vi "ColourROIPicker.vi"() -> ()   [LabVIEW 2021]
uses:
  <vilib>/userDefined/High Color/IMAQdx.ctl
  <vilib>/vision/driver/IMAQdx.llb/IMAQdx Camera Control Mode.ctl
  <vilib>/vision/driver/IMAQdx.llb/IMAQdx Acquisition Mode.ctl
  <vilib>/vision/driver/IMAQdx.llb/IMAQdx Buffer Number Mode.ctl
  <vilib>/vision/driver/NI_Vision_Acquisition_Software.lvlib
  <resource>/objmgr/imaqdx.rc
  <vilib>/vision/NI_Vision_Development_Module.lvlib
panel:
  out "Is Colour from Sample Detected":bool
  out "Colour at Pixel Box":u32(colorbox)
  out "Colour at Pixel Value":u32
  out "Model":string
  out "Attr":T1(array[cluster]) caption="Camera Attributes"
  out "Image":T2(plugin-control)
  in  "Stop":bool
  out "error out":errorcluster
  # "RPV Test Rig 2024"
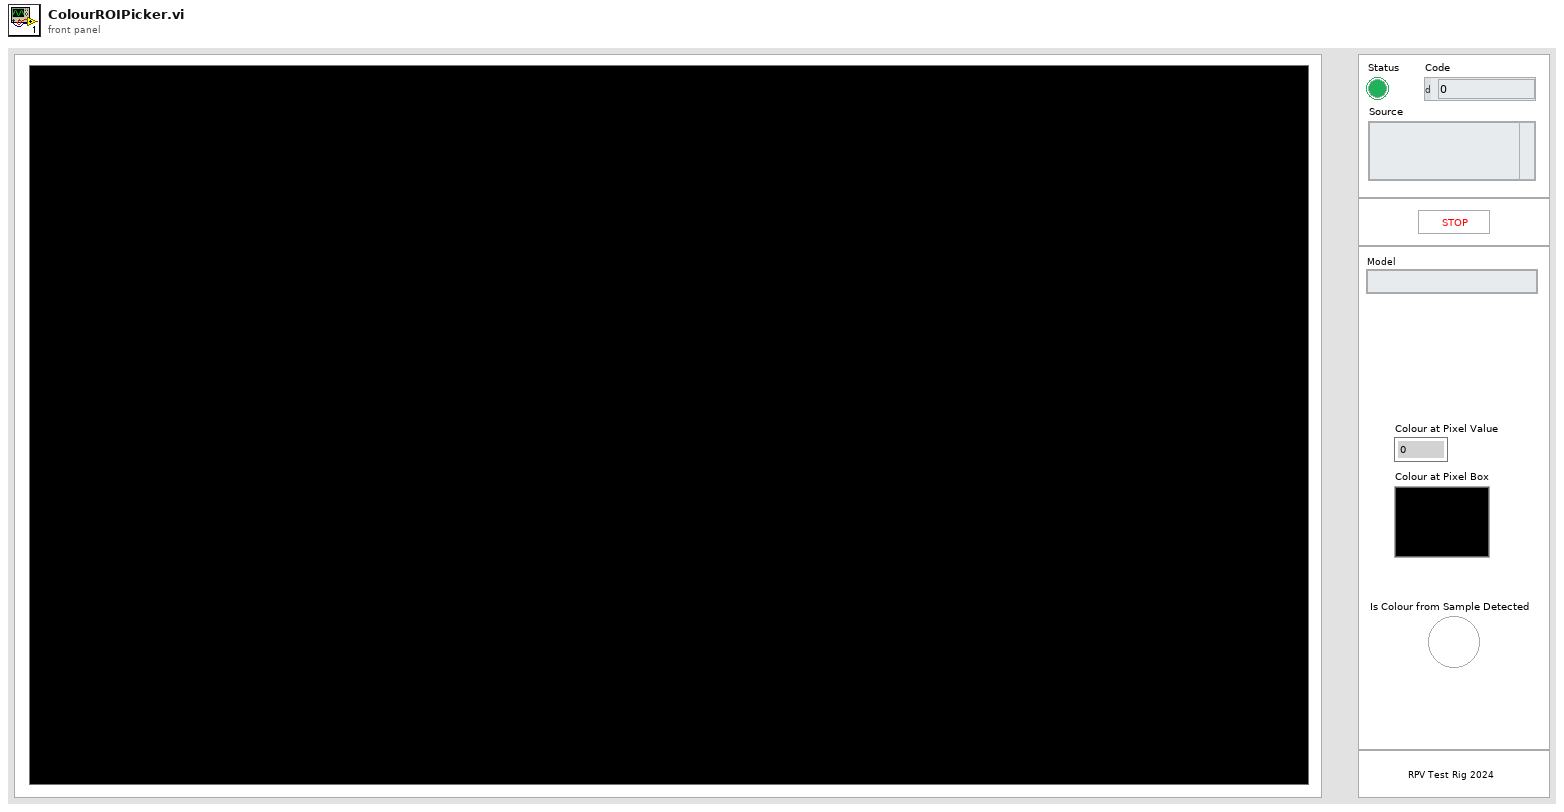
[diagram p1: front panel]
types:
  T1 = cluster{"Data Type":enum32{"U32", "I64", "DBL", "String", "Enum", "Bool", "Command"}, "Readable":bool, "Writable":bool, "Attribute Name":string}[]
  T2 = typedef "IMAQ Image.ctl" = refnum<image>
  T3 = typedef "IMAQ Rectangle" = cluster{"Left":i32, "Top":i32, "Right":i32, "Bottom":i32, "Rotation":dbl}
  T4 = typedef "NI_Vision_Acquisition_Software.lvlib/IMAQdx Buffer Number Mode.ctl" = enum32{"Next", "Last", "Buffer Number", "Every", "Last New"}
  T5 = typedef "NI_Vision_Acquisition_Software.lvlib/IMAQdx Acquisition Mode.ctl" = enum32{"One Shot", "Continuous"}
  T6 = typedef "NI_Vision_Acquisition_Software.lvlib/IMAQdx Camera Control Mode.ctl" = enum32{"Controller", "Listener"}
  T7 = typedef "IMAQdx.ctl" = refnum<k21>
  T8 = typedef "ROI Descriptor" = cluster{"Global Rectangle":i32[], "Contours":cluster{"ID":enum32{"External", "Internal"}, "Type":u32, "Coordinates":i32[]}[]}
  T9 = typedef "NI_Vision_Acquisition_Software.lvlib/IMAQdx Attribute Type.ctl" = enum32{"U32", "I64", "DBL", "String", "Enum", "Bool", "Command"}
  T10 = cluster{"Attribute Type":T9, "Readable":bool, "Writable":bool, "Attribute Name":string}[]
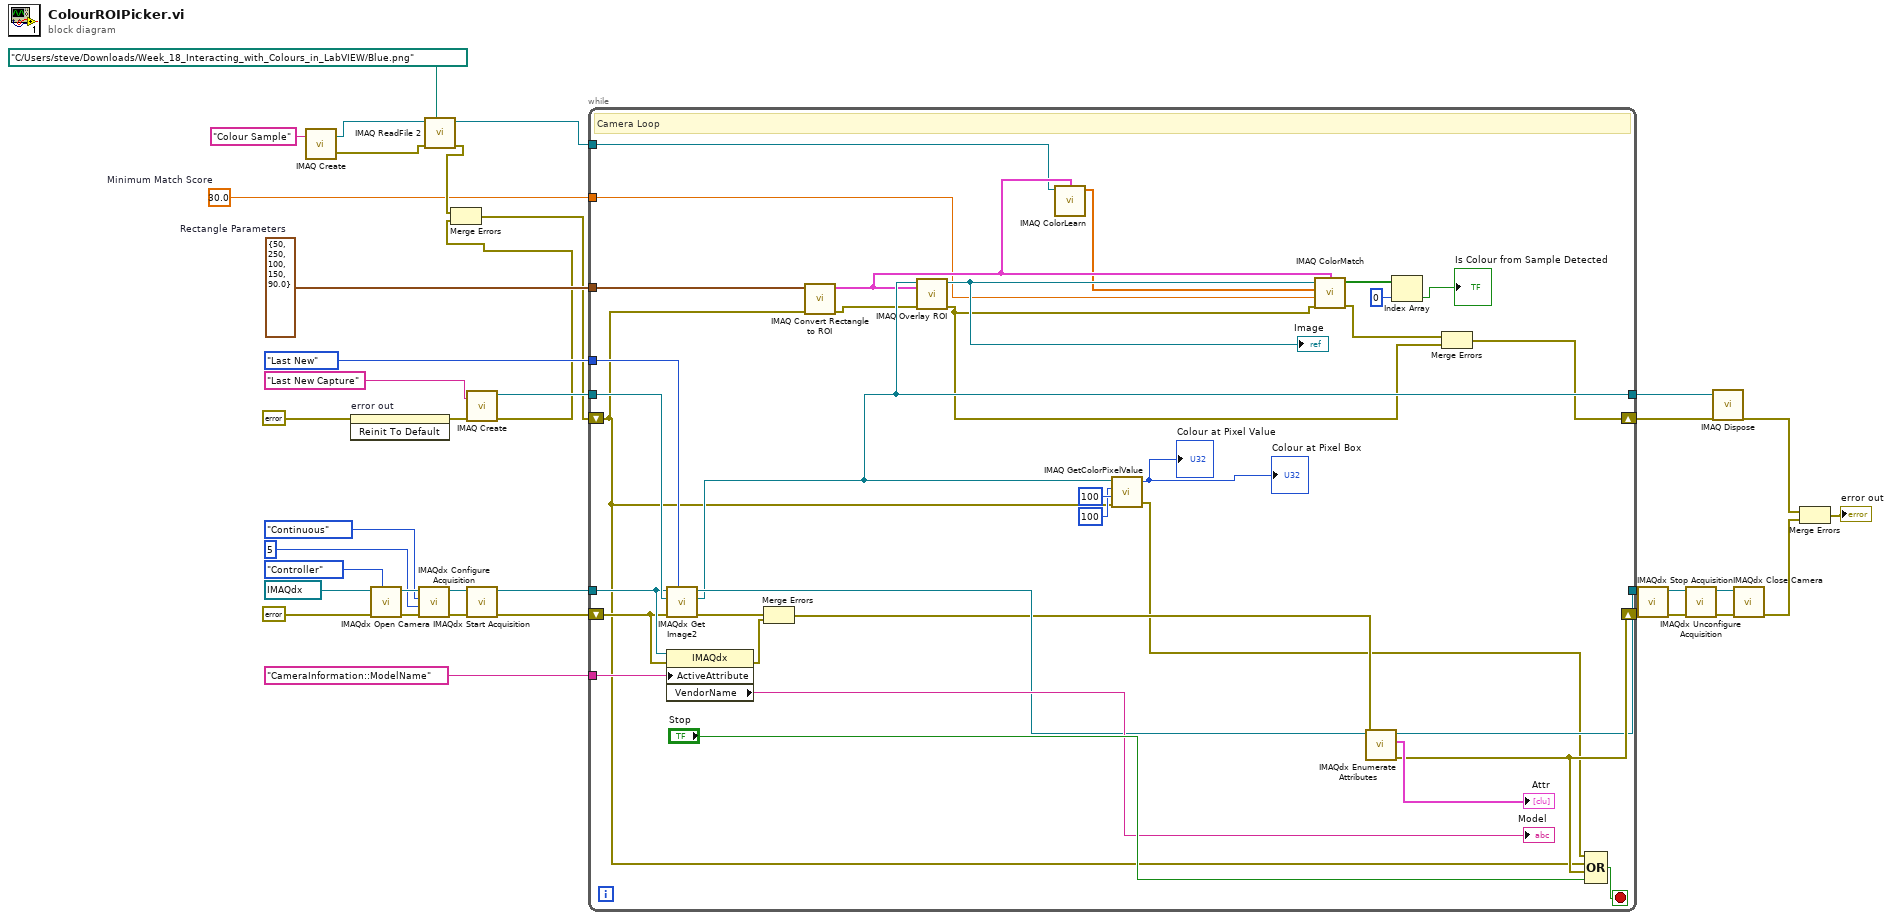
[diagram p0: block diagram]
diagram:
  w1 = 30.0  # Minimum Match Score
  w10 = T3 {"Left"=50, "Top"=250, "Right"=100, "Bottom"=150, "Rotation"=90.0}  # Rectangle Parameters
  n1 = call "IMAQ Create"("Image Name"="Colour Sample") -> ("New Image"=w5:T2, "error out"=w3:errorcluster)  [unwired: 4 in]
  n2 = invoke on="error out" class="Clust (strict)" method="Reinit To Default"(error in=errorcluster {"status"=FALSE, "code"=0, "source"=""}) -> (error out=w13:errorcluster)  [unwired: 2 in, 2 out]
  n3 = call <vilib>:"IMAQdx Open Camera.vi"("Camera Control Mode"=IMAQdx_Camera_Control_Mode."Controller", "error in"=errorcluster {"status"=FALSE, "code"=0, "source"=""}, "Session In"=T7 "cam0") -> ("error out"=w38:errorcluster, "Session Out"=w37:T7)  [unwired: 7 in]
  n4 = call <vilib>:"IMAQdx Configure Acquisition.vi"("error in"=w38, "Number of Buffers"=u32 5, "Continuous?"=IMAQdx_Acquisition_Mode."Continuous", "Session In"=w37) -> ("error out"=w32:errorcluster, "Session Out"=w31:T7)  [unwired: 6 in]
  n5 = call "IMAQ ReadFile 2"("File Path"=path "C:/Users/steve/Downloads/Week_18_Interacting_with_Colours_in_LabVIEW/Blue.png", "error in (no error)"=w3, "Image"=w5) -> ("error out"=w2:errorcluster, "Image Out"=w4:T2)  [unwired: 4 in, 3 out]
  n6 = call "IMAQ Create"("Image Name"="Last New Capture", "error in (no error)"=w13) -> ("New Image"=w20:T2, "error out"=w8:errorcluster)  [unwired: 3 in]
  n7 = Merge Errors(w2, w8) -> (w7:errorcluster)
  n8 = call <vilib>:"IMAQdx Start Acquisition.vi"("error in"=w32, "Session In"=w31) -> ("error out"=w25:errorcluster, "Session Out"=w23:T7)  [unwired: 8 in]
  n9 = while {
    shift-right: [w65] -> w24
    shift-left: w25 -> [w62]
    tunnel: w23 -> [w63]
    tunnel: [w64] -> w22
    tunnel: IMAQdx_Buffer_Number_Mode."Last New" ("Buffer Number Mode (Next)") -> [w72]
    shift-right: [w40] -> w17
    shift-left: w7 -> [w46]
    tunnel: w20 -> [w71]
    tunnel: [w52] -> w18
    tunnel: "CameraInformation::ModelName" ("ActiveAttribute") -> [w67]
    tunnel: w10 -> [w53]
    tunnel: w4 -> [w47]
    tunnel: w1 -> [w39]
    stop <- w69 stop-if-true
    # "Camera Loop"
    n10 = call <vilib>:"IMAQdx Get Image2.vi"("Buffer Number Mode (Next)"=w72, "error in"=w62, "Image In"=w71, "Session In"=w63) -> ("error out"=w61:errorcluster, "Image Out"=w52:T2, "Session Out"=w59:T7)  [unwired: 4 in, 1 out]
    n11 = property class="IMAQdx"(reference=w63, error in=w62, "ActiveAttribute"=w67) -> (error out=w60:errorcluster, "VendorName"=→"Model":string)  [unwired: 1 out]
    n12 = Merge Errors(w61, w60) -> (w58:errorcluster)
    n13 = call "IMAQ Convert Rectangle to ROI"("error in (no error)"=w46, "Rectangle"=w53) -> ("error out"=w51:errorcluster, "ROI Descriptor"=w49:T8)  [unwired: 7 in]
    n14 = call "IMAQ Overlay ROI"("error in (no error)"=w51, "ROI Descriptor"=w49, "Image"=w52) -> ("error out"=w41:errorcluster, "Image Out"=w50:T2)  [unwired: 7 in]
    "Image" <- w50
    n15 = call "IMAQ ColorLearn"("ROI Descriptor"=w49, "Image"=w47) -> ("Color Spectrum"=w48:dbl[])  [unwired: 6 in, 1 out]
    n16 = call "IMAQ GetColorPixelValue"("error in (no error)"=w46, "Y Coordinate"=100, "X Coordinate"=100, "Image"=w52) -> ("error out"=w55:errorcluster, "Pixel Value (U32)"=→"Colour at Pixel Value" →"Colour at Pixel Box":u32)  [unwired: 1 out]
    n17 = call "IMAQ ColorMatch"("ROI Descriptor"=w49, "Image"=w50, "Color Spectrum"=w48, "Minimum Match Score"=w39, "error in (no error)"=w41) -> ("Match Flag"=w45:bool[], "error out"=w42:errorcluster)  [unwired: 2 in, 1 out]
    n18 = call <vilib>:"IMAQdx Enumerate Attributes.vi"("error in"=w58, "Session In"=w59) -> ("error out"=w65:errorcluster, "Attribute Information Array"=→"Attr":T10, "Session Out"=w64:T7)  [unwired: 7 in]
    n19 = Index Array(array=w45, index=0) -> (element=→"Is Colour from Sample Detected":bool)
    n20 = Merge Errors(w42, w41) -> (w40:errorcluster)
    n21 = Compound Arithmetic op=OR(w55, w46, w65, "Stop") -> (w69:bool)
  }
  n22 = call <vilib>:"IMAQdx Stop Acquisition.vi"("error in"=w24, "Session In"=w22) -> ("error out"=w34:errorcluster, "Session Out"=w33:T7)  [unwired: 8 in]
  n23 = call <vilib>:"IMAQdx Unconfigure Acquisition.vi"("error in"=w34, "Session In"=w33) -> ("error out"=w36:errorcluster, "Session Out"=w35:T7)  [unwired: 8 in]
  n24 = call "IMAQ Dispose"("Image"=w18, "error in (no error)"=w17) -> ("error out"=w15:errorcluster)  [unwired: 4 in]
  n25 = call <vilib>:"IMAQdx Close Camera.vi"("error in"=w36, "Session In"=w35) -> ("error out"=w14:errorcluster)  [unwired: 9 in]
  n26 = Merge Errors(w15, w14) -> (→"error out":errorcluster)
